vi "LVClass_ComputePhaseSet dtor.vi"(0 "ComputePhaseSet in":refnum<class "ComputePhaseSet.lvclass">, 11 "error in (no error)":errorcluster) -> (4 "ComputePhaseSet out":refnum<class "ComputePhaseSet.lvclass">, 15 "error out":errorcluster)   [LabVIEW 2020, in "ComputePhaseSet.lvclass"]
doc: "ComputePhaseSet Destructor.\n\n--------------------------------------------------------------------------------\n\n<B>ComputePhaseSetIn </B> : ComputePhaseSet object.\n<B>ComputePhaseSetOut </B> : ComputePhaseSet object.\n<B>ErrorIn </B> : Error\n<B>ErrorOut </B> : Error\n\n--------------------------------------------------------------------------------"
uses:
  ComputePhaseSet.lvclass
  ComputePhaseSet.lvclass/ComputePhaseSet.ctl
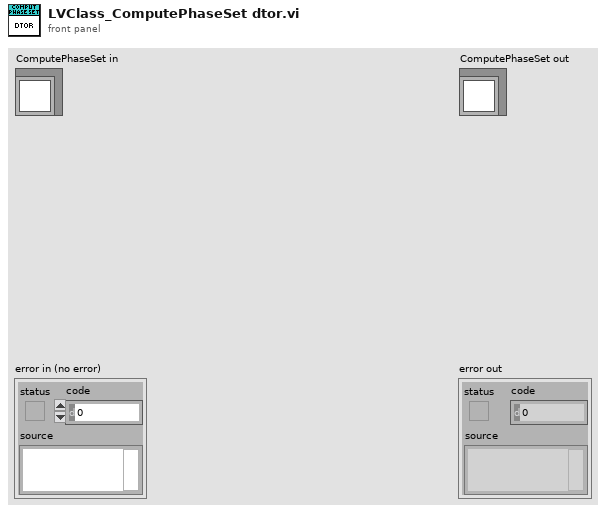
[diagram p1: front panel]
types:
  T1 = typedef "Handle creation.ctl" = enum16{"By ctor", "By write function"}
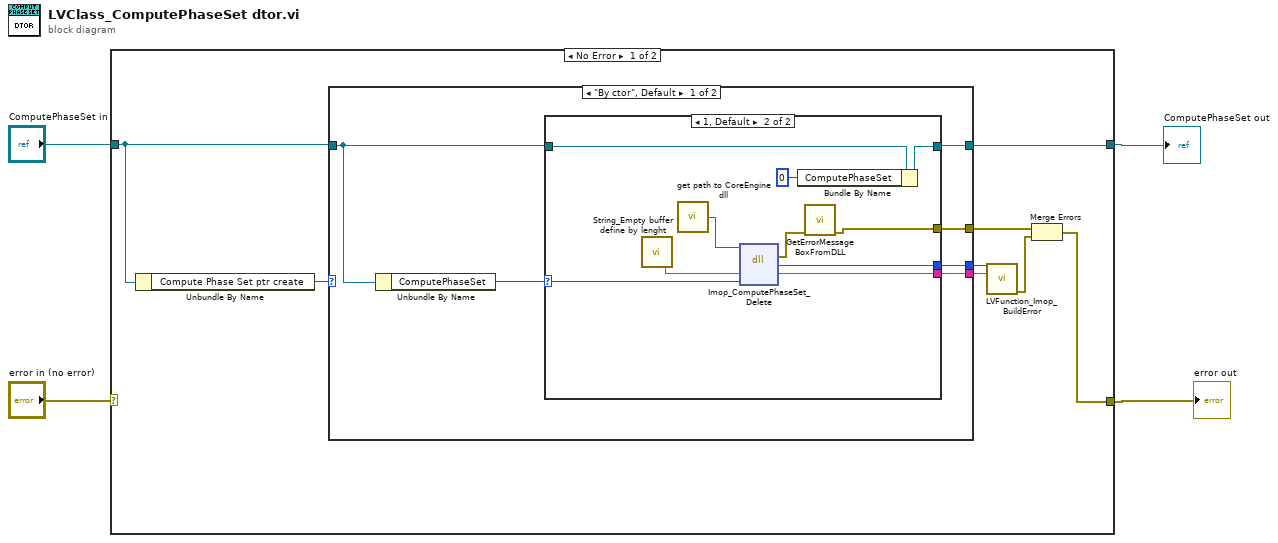
[diagram p0: block diagram]
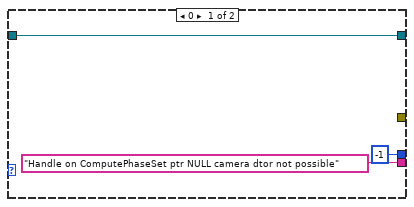
[diagram p2: hidden frame]
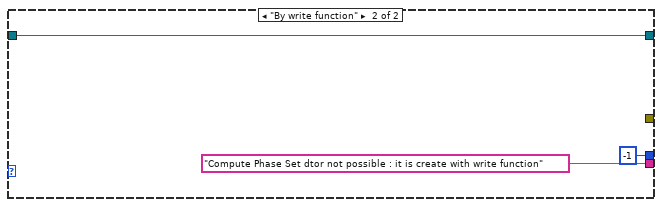
[diagram p3: hidden frame]
diagram:
  n1 = case shown="No Error" "error in (no error)" {
    selector: "error in (no error)" -> [_ w36]
    tunnel: [w5 w36] -> w1
    tunnel: [w10 w35] -> w2
    tunnel: "ComputePhaseSet in" -> [w9 w35]
    frame No Error {
      n2 = Unbundle By Name(w9) -> ("Compute Phase Set ptr create"=w8:T1)
      n3 = case shown="\"By ctor\", Default" w8 {
        tunnel: [w18 w34] -> w10
        tunnel: [w17 -1] -> w12
        tunnel: [w16 "Compute Phase Set dtor not possible : it is create with write function" ("message")] -> w11
        tunnel: w9 -> [w15 w34]
        tunnel: [w13 _] -> w7
        frame "By ctor", Default {
          n4 = Unbundle By Name(w15) -> ("ComputePhaseSet"=w14:i32)
          n5 = case shown="1, Default" w14 {
            selector: w14 -> [_ w28]
            tunnel: w15 -> [w21 w31]
            tunnel: [w21 w30] -> w18
            tunnel: [-1 w26] -> w17
            tunnel: ["Handle on ComputePhaseSet ptr NULL camera dtor not possible" ("message") w27] -> w16
            tunnel: [_ w22] -> w13
            frame 0 {
            }
            frame 1, Default {
              n6 = call "String_Empty buffer define by lenght.vi"() -> ("Empty buffer"=w29:string)  [unwired: 1 in]
              n7 = call "get path to CoreEngine dll.vi"() -> ("path to c_interface_vc100.dll"=w25:path)  [unwired: 12 in, 3 out]
              n8 = dll-call lib="D:/soft/HASO_v3/SVN_trunk/ImOpCoreEngine4_LV2011/DLLs/c_interface_vc100.dll" fn="Imop_ComputePhaseSet_Delete"(path in=w25, "message"=w29, "objet"=w28) -> (error out=w24:errorcluster, "return type"=w26:i32, "message"=w27:string)  [unwired: 3 in, 1 out]
              n9 = Bundle By Name(cluster=w31, "ComputePhaseSet"=0) -> (w30:refnum<class "ComputePhaseSet.lvclass">)
              n10 = call "GetErrorMessageBoxFromDLL.vi"("error IN"=w24) -> ("error OUT"=w22:errorcluster)  [unwired: 10 in]
            }
          }
        }
        frame "By write function" {
        }
      }
      n11 = call "LVFunction_Imop_BuildError.vi"("code"=w12, "String to Prepend to source (\"\")"=w11) -> ("error out"=w6:errorcluster)  [unwired: 13 in]
      n12 = Merge Errors(w7, w6) -> (w5:errorcluster)
    }
    frame Error {
    }
  }
  "error out" <- w1
  "ComputePhaseSet out" <- w2
